vi "UsrProfiles-Validate copied profile path.vi"(8 "error in":errorcluster) -> (0 "error out":errorcluster, 1 "Copied profile file path":path, 3 "copied profile file still exists":bool)   [LabVIEW 2013]
uses:
  Globals/gl_UsrProfiles globals.vi
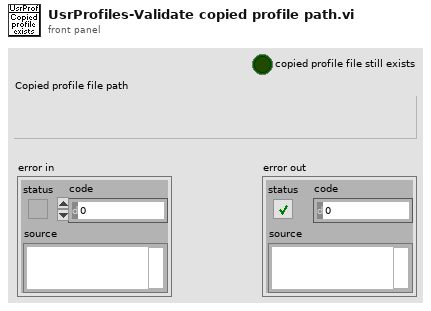
[diagram p1: front panel]
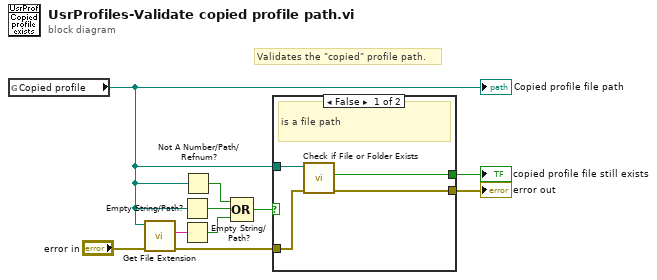
[diagram p0: block diagram]
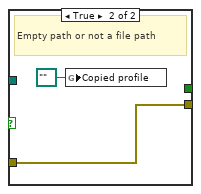
[diagram p2: hidden frame]
diagram:
  # "Validates the \"copied\" profile path."
  n1 = global read "gl_UsrProfiles globals.vi" "Copied profile"() -> (w8:path)
  "Copied profile file path" <- w8
  n2 = call <vilib>:"Get File Extension.vi"("error in (no error)"="error in", "file"=w8) -> ("error out"=w7:errorcluster, "lowercase file extension"=w3:string)  [unwired: 6 in, 2 out]
  n3 = Empty String/Path?(string/path=w8) -> (empty?=w4:bool)
  n4 = Empty String/Path?(string/path=w3) -> (empty?=w5:bool)
  n5 = Not A Number/Path/Refnum?(number/path/refnum=w8) -> (NaN/Path/Refnum?=w9:bool)
  n6 = Compound Arithmetic op=OR(w9, w4, w5) -> (w6:bool)
  n7 = case shown="False" w6 {
    tunnel: w8 -> [w14 _]
    tunnel: w7 -> [w13 w15]
    tunnel: [w12 _] -> w10
    tunnel: [w11 w15] -> w2
    frame False {
      # "is a file path"
      n8 = call <vilib>:"Check if File or Folder Exists.vi"("error in (no error)"=w13, "path"=w14) -> ("error out"=w11:errorcluster, "file or folder exists?"=w12:bool)  [unwired: 7 in, 1 out]
    }
    frame True {
      # "Empty path or not a file path"
      n9 = global write "gl_UsrProfiles globals.vi" "Copied profile"(path "" ("Copied profile")) -> ()
    }
  }
  "copied profile file still exists" <- w10
  "error out" <- w2
